vi "Sequence.GetSequenceChannels.vi"(6 "Refs":refnum<vi>[](array[refnum]), 8 "error in (no error)":errorcluster, 9 "Aliases Array":string[](array[string]), 10 "Aliases.All":T1[](array[typedef]), 11 "ChannelsLookup":variant) -> (0 "error out":errorcluster, 2 "SequenceChannels":T2, 3 "ChannelsLookup":variant)   [LabVIEW 2013, in "Simple Sequence Editor.lvlib"]
uses:
  Simple Sequence Editor.lvlib
  Types/Compiled.SequenceChannels.ctl
  Types/ChannelProperties.ctl
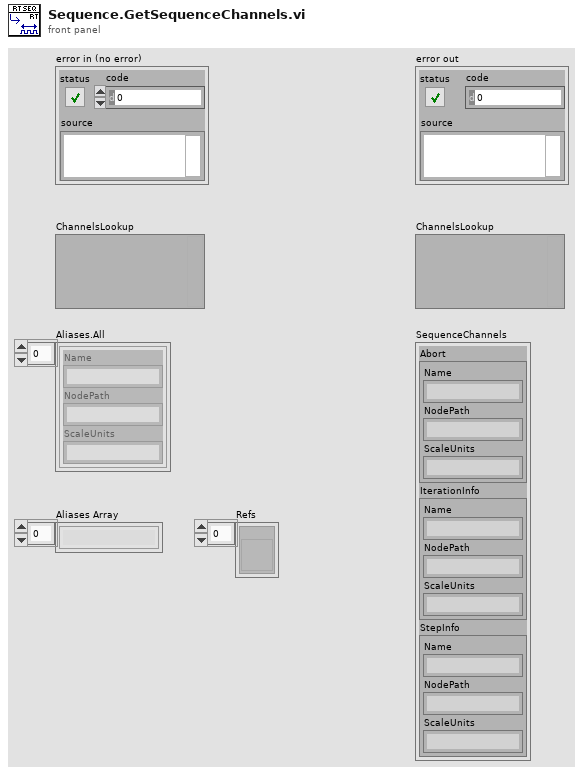
[diagram p1: front panel]
types:
  T1 = typedef "Simple Sequence Editor.lvlib/ChannelProperties.ctl" = cluster{"Name":string, "NodePath":string, "ScaleUnits":string}
  T2 = typedef "Simple Sequence Editor.lvlib/Compiled.SequenceChannels.ctl" = cluster{"Abort":T1, "IterationInfo":T1, "StepInfo":T1}
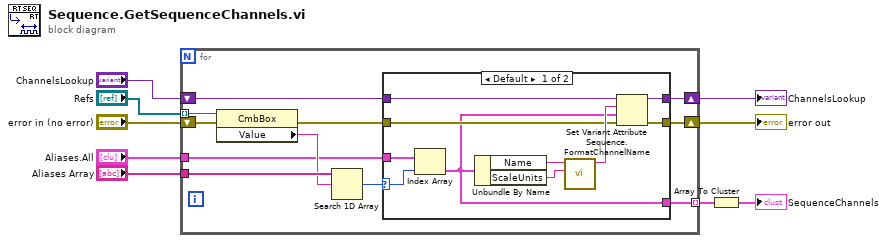
[diagram p0: block diagram]
diagram:
  n1 = for {
    tunnel: "Refs" -> [w19] mode=indexing
    shift-right: [w13] -> w1
    shift-left: "error in (no error)" -> [w20]
    tunnel: "Aliases.All" -> [w15]
    tunnel: "Aliases Array" -> [w18]
    shift-right: [w11] -> w9
    shift-left: "ChannelsLookup" -> [w12]
    tunnel: [w10] -> w5 mode=indexing
    n2 = property class="CmbBox"(reference=w19, error in=w20) -> (error out=w14:errorcluster, "Value"=w17:string)  [unwired: 1 out]
    n3 = Search 1D Array(1D array=w18, element=w17) -> (index of element=w16:i32)  [unwired: 1 in]
    n4 = case shown="Default" w16 {
      selector: w16 -> [w29 _]
      tunnel: w15 -> [w30 _]
      tunnel: w14 -> [w25 w31]
      tunnel: [w24 w31] -> w13
      tunnel: w12 -> [w23 w32]
      tunnel: [w22 w32] -> w11
      tunnel: [w21 _] -> w10
      frame Default {
        n5 = Index Array(array=w30, index=w29) -> (element=w21:T1)
        n6 = Unbundle By Name(w21) -> ("Name"=w27:string, "ScaleUnits"=w26:string)
        n7 = call "Sequence.FormatChannelName.vi"("ScaleUnits"=w26, "Name"=w27) -> ("String"=w28:string)  [unwired: 9 in]
        n8 = Set Variant Attribute(Variant=w23, name=w28, value=w21, error in=w25) -> (Variant out=w22:variant, error out=w24:errorcluster)  [unwired: 1 out]
      }
      frame -1 {
      }
    }
  }
  "ChannelsLookup" <- w9
  "error out" <- w1
  n9 = Array To Cluster(array=w5) -> (cluster=→"SequenceChannels":cluster{"[0]":T1, "[1]":T1, "[2]":T1})
